vi "Build UBX Message.vi"(6 "Payload":i8[](array[numeric]), 7 "Class":i8 format="%x", 8 "error in":errorcluster, 9 "Length":i8[](array[numeric]), 10 "ID":i8 format="%x", 11 "VISA resource name":refnum<visa-resource-name>) -> (0 "error out":errorcluster, 2 "UBX Message":string, 3 "VISA resource name out":refnum<visa-resource-name>)   [LabVIEW 2011, in "u-blox 5 Series.lvlib"]
doc: "Builds Class, ID, Length, and Payload into a UBX Sentence. See the UBX Protocol Specifications for more details."
uses:
  u-blox 5 Series.lvlib
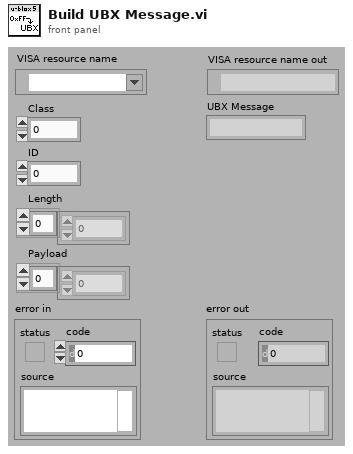
[diagram p1: front panel]
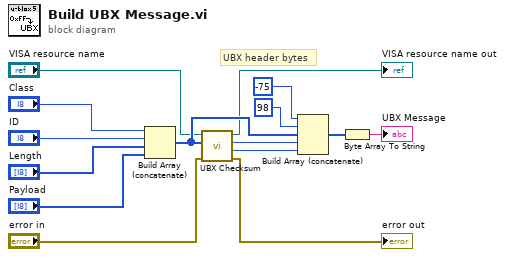
[diagram p0: block diagram]
diagram:
  # "UBX header bytes"
  n1 = Build Array (concatenate)("Class", "ID", "Length", "Payload") -> (w13:i8[])
  n2 = call "UBX Checksum.vi"("error in"="error in", "Checksum Packet"=w13, "VISA resource name"="VISA resource name") -> ("error out"=→"error out":errorcluster, "CK_B"=w15:i8, "CK_A"=w14:i8, "VISA resource name out"=→"VISA resource name out":refnum<visa-resource-name>)  [unwired: 5 out]
  n3 = Build Array (concatenate)(i8 -75, i8 98, w13, w14, w15) -> (w11:i8[])
  n4 = Byte Array To String(unsigned byte array=w11) -> (string=→"UBX Message":string)
